vi "Set_Source.vi"(6 "Source Status":T7, 7 "Establish Exp Conditions":bool, 8 "Traverse line":T3 {"Row Duration (mins)" format="%#.1f"; "Row No" min=0; "Trace Gas Concentration (%)" min=0.0 format="%#.2f"; "Emission Rate (l/min)" format="%#.2f"; "Tunnel Speed" format="%#.2f"; "Start X" format="%#.2f"; "Start Y" format="%#.2f"; "Start Z" format="%#.2f"; "End X" format="%#.2f"; "End Y" format="%#.2f"; "End Z" format="%#.2f"; "Averaging time (min)" min=0.0 format="%#.1f"}, 9 "Simulate/Run":T6) -> (0 "Status Cluster":T1, 1 "Flowrates (kg/min)":dbl[](array[numeric]) format="%.2f", 2 "Time Source Started":dbl, 3 "Flowrates Achieved?":bool, 4 "Source requested?":bool, 5 "Source Est Time":dbl format="%.2f")   [LabVIEW 2010]
uses:
  ADAM Client/Sub VIs/ADAM Controls/Client_Source_Status.ctl
  Controls/User_Specific_mode.ctl
  Traverse_cluster.ctl
  Spacing.ctl
  Controls/Multi_run_mode.ctl
  Status_Cluster.ctl
  Multi_Run_Status.ctl
  Globals/Trav_pos_global.vi
  Globals/Extra_Commands_Global.vi
panel:
  # "X           Y            Z"
  # "Start"
  # "End"
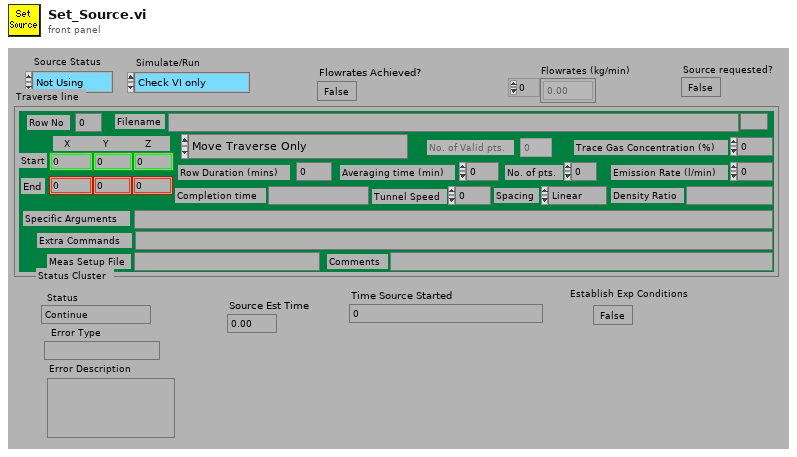
[diagram p1: front panel]
types:
  T1 = typedef "Status_Cluster.ctl" = cluster{"Status":T2, "Error Type":string, "Error Description":string}
  T2 = typedef "Multi_Run_Status.ctl" = enum16{"Continue", "Jump to Next Point", "Jump to Next Row", "Jump To Fall Back", "Terminate Run"}
  T3 = typedef "Traverse_cluster.ctl" = cluster{"Start X":dbl, "Start Y":dbl, "Start Z":dbl, "End X":dbl, "End Y":dbl, "End Z":dbl, "No. of pts.":i32, "Spacing":T4, "Filename":path, "Tunnel Speed":dbl, "Averaging time (min)":dbl, "Extra Commands":string, "Specific Arguments":string, "Emission Rate (l/min)":dbl, "Trace Gas Concentration (%)":dbl, "Density Ratio":string, "Comments":string, "Row No":i32, "Row Type Selector":T5, "Completion time":string, "Row Duration (mins)":dbl, "No. of Valid pts.":i32, "Meas Setup File":string}
  T4 = typedef "Spacing.ctl" = enum16{"Linear", "Log", "Gauss", "Specified", "N/A"}
  T5 = typedef "Multi_run_mode.ctl" = enum16{"Move Traverse Only", "Set Tunnel Speed Only", "Set Source Only", "Set Measurement Conditions", "Single Measurement", "Vertical Profile", "Lateral Profile", "Longitudinal Profile", "Explore Volume", "Multi-Axis Profile", "Auto Calibrate", "Meas Fast FID Bkgnd", "Check Beam Power", "Scanning Valve Measurement", "Run VI Named:", "Set ADAM Ch", "Wait (minutes)", "Send Message", "Synchronize With:", "Fall Back to this Row", "Turn Off Row Repeating", "Blank Row"}
  T6 = typedef "User_Specific_mode.ctl" = enum16{"Check VI only", "Run VI"}
  T7 = typedef "Client_Source_Status.ctl" = enum16{"Not Using", "Using", "Must Have"}
  T8 = cluster{"Emission Rate (l/min)":dbl, "Trace Gas Concentration (%)":dbl, "Density Ratio":string}
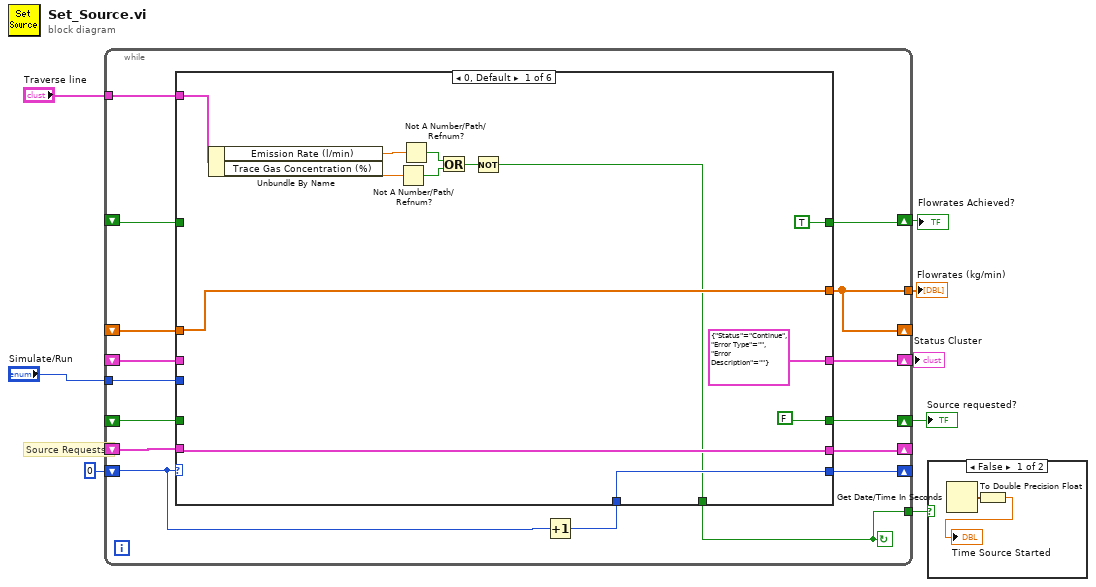
[diagram p0: block diagram]
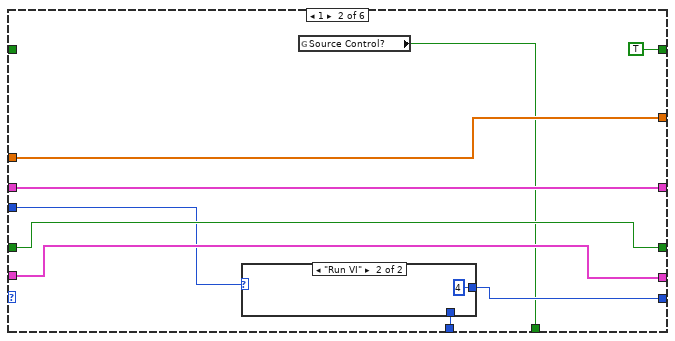
[diagram p3: hidden frame]
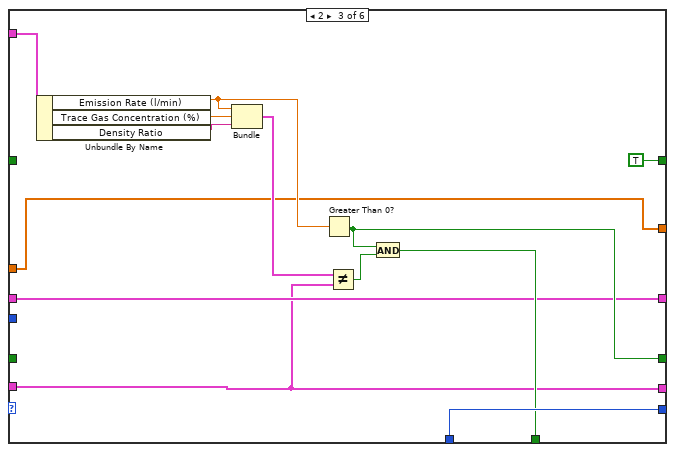
[diagram p5: hidden frame]
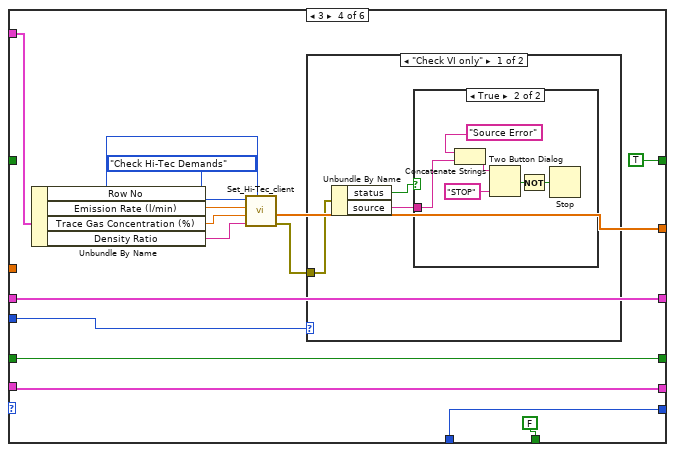
[diagram p6: hidden frame]
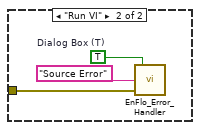
[diagram p8: hidden frame]
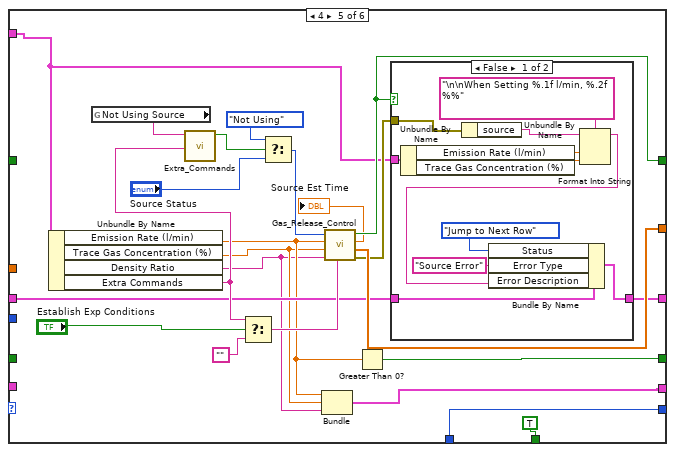
[diagram p9: hidden frame]
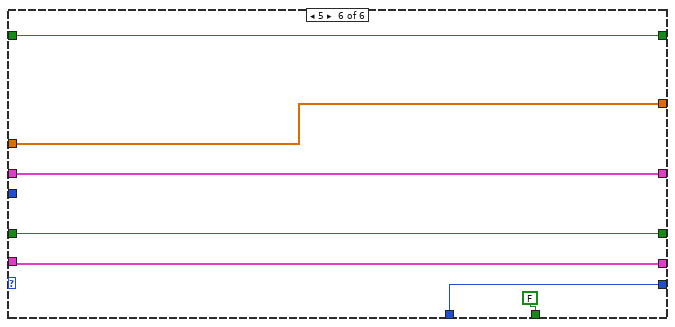
[diagram p11: hidden frame]
diagram:
  # "Source Requests"
  n1 = while {
    shift-left: _ -> [w12]
    shift-right: [w13] -> w4
    shift-left: _ -> [w14]
    shift-right: [w15] -> w5
    shift-left: _ -> [w16]
    shift-right: [w19] -> w6
    shift-left: 0 -> [w18]
    shift-right: [w20] -> _
    shift-left: _ -> [w21]
    shift-right: [w22] -> _
    tunnel: [w22] -> w8
    shift-left: _ -> [w24]
    shift-right: [w23] -> _
    tunnel: "Simulate/Run" -> [w11]
    tunnel: "Traverse line" -> [w10]
    tunnel: [w9] -> w1
    stop <- w9 continue-if-true
    n2 = Increment(x=w18) -> (x+1=w17:i32)
    n3 = case shown="0, Default" w18 {
      tunnel: [w35 w46 w52 w71 w102 w125] -> w22
      tunnel: w24 -> [w32 w44 w50 w68 _ w129]
      tunnel: [w32 w44 w50 w68 w91 w129] -> w23
      tunnel: w21 -> [w35 w46 w52 _ _ w125]
      tunnel: [FALSE w40 w61 w69 w111 w130] -> w19
      tunnel: [TRUE ("Flowrates Achieved?") TRUE ("Flowrates Achieved?") TRUE ("Flowrates Achieved?") TRUE ("Flowrates Achieved?") w103 w124] -> w13
      tunnel: [w25 w38 w55 FALSE TRUE FALSE] -> w9
      tunnel: [w31 w43 w56 w67 w100 w128] -> w20
      tunnel: w17 -> [w31 w41 w56 w67 w100 w128]
      tunnel: w16 -> [_ w40 _ w69 _ w130]
      tunnel: [T1 {"Status"=enum."Continue", "Error Type"="", "Error Description"=""} ("Status Cluster") w42 w51 w65 w101 w126] -> w15
      tunnel: w14 -> [_ w42 w51 w65 w95 w126]
      tunnel: w12 -> [_ _ _ _ _ w124]
      tunnel: w11 -> [_ w39 _ w63 _ _]
      tunnel: w10 -> [w29 _ w49 w62 w89 _]
      frame 0, Default {
        n4 = Unbundle By Name(w29) -> ("Emission Rate (l/min)"=w37:dbl, "Trace Gas Concentration (%)"=w30:dbl)
        n5 = Not A Number/Path/Refnum?(number/path/refnum=w30) -> (NaN/Path/Refnum?=w28:bool)
        n6 = Not A Number/Path/Refnum?(number/path/refnum=w37) -> (NaN/Path/Refnum?=w27:bool)
        n7 = Or(x=w27, y=w28) -> (x .or. y?=w26:bool)
        n8 = Not(x=w26) -> (.not. x?=w25:bool)
      }
      frame 1 {
        n9 = case shown="\"Run VI\"" w39 {
          tunnel: [w47 4] -> w43
          tunnel: w41 -> [w47 _]
          frame "Check VI only" {
          }
          frame "Run VI" {
          }
        }
        n10 = global read "Trav_pos_global.vi" "Source Control?"() -> (w38:bool)
      }
      frame 2 {
        n11 = Unbundle By Name(w49) -> ("Emission Rate (l/min)"=w58:dbl, "Trace Gas Concentration (%)"=w60:dbl, "Density Ratio"=w59:string)
        n12 = Bundle("Emission Rate (l/min)"=w58, "Trace Gas Concentration (%)"=w60, "Density Ratio"=w59) -> (w54:T8)  [unwired: 1 out]
        n13 = Greater Than 0?(x=w58) -> (x > 0?=w61:bool)
        n14 = Not Equal?(x=w54, y=w50) -> (x != y?=w57:bool)
        n15 = And(x=w61, y=w57) -> (x .and. y?=w55:bool)
      }
      frame 3 {
        n16 = Unbundle By Name(w62) -> ("Row No"=w72:i32, "Emission Rate (l/min)"=w75:dbl, "Trace Gas Concentration (%)"=w74:dbl, "Density Ratio"=w73:string)
        n17 = call "Set_Hi-Tec_client.vi"("Row No"=w72, "Density Ratio"=w73, "Strength (% by volume)"=w74, "Stack flowrate (l/min)"=w75, "Mode"=enum16{"Control Hi-Tec", "Check Hi-Tec Demands"}."Check Hi-Tec Demands") -> ("error out"=w64:errorcluster, "Flowrates (kg/min)"=w71:dbl[])  [unwired: 3 out]
        n18 = case shown="\"Check VI only\"" w63 {
          tunnel: w64 -> [w79 w88]
          frame "Check VI only" {
            n19 = Unbundle By Name(w79) -> ("status"=w77:bool, "source"=w78:string)
            n20 = case shown="True" w77 {
              tunnel: w78 -> [_ w84]
              frame False {
              }
              frame True {
                n21 = Concatenate Strings("Source Error" ("Error Type"), w84) -> (w83:string)
                n22 = Two Button Dialog(message=w83, 1:"STOP" ("F button name (\"Cancel\")")) -> (T button?=w81:bool)  [unwired: 1 out]
                n23 = Not(x=w81) -> (.not. x?=w80:bool)
                n24 = Stop(stop? (T)=w80) -> ()
              }
            }
          }
          frame "Run VI" {
            w86 = TRUE  # Dialog Box (T)
            n25 = call "EnFlo_Error_Handler.vi"("error in (no error)"=w88, "Error Type"="Source Error", "Dialog Box (T)"=w86) -> ()  [unwired: 3 out]
          }
        }
      }
      frame 4 {
        n26 = Unbundle By Name(w89) -> ("Emission Rate (l/min)"=w94:dbl, "Trace Gas Concentration (%)"=w93:dbl, "Density Ratio"=w92:string, "Extra Commands"=w105:string)
        n27 = global read "Extra_Commands_Global.vi" "Not Using Source"() -> (w108:string)
        n28 = call "Extra_Commands.vi"("String to Search"=w105, "Command"=w108) -> ("Command Found"=w107:bool)  [unwired: 1 in, 4 out]
        n29 = Select(t=w105, s="Establish Exp Conditions", f="") -> (s? t:f=w104:string)
        n30 = Select(t=Client_Source_Status."Not Using" ("Source Status"), s=w107, f="Source Status") -> (s? t:f=w106:T7)
        n31 = Bundle("Emission Rate (l/min)"=w94, "Trace Gas Concentration (%)"=w93, "Density Ratio"=w92) -> (w91:T8)  [unwired: 1 out]
        n32 = call "Gas_Release_Control.vi"("Extra Commands"=w104, "Density Ratio"=w92, "Strength (% by volume)"=w93, "Stack flowrate (l/min)"=w94, "Source Status"=w106) -> ("error out"=w90:errorcluster, "Flowrates (kg/min)"=w102:dbl[], "Source Est Time (s)"=→"Source Est Time":dbl, "Flowrates Achieved?"=w103:bool)  [unwired: 1 out]
        n33 = Greater Than 0?(x=w94) -> (x > 0?=w111:bool)
        n34 = case shown="False" w103 {
          tunnel: [w118 w123] -> w101
          tunnel: w95 -> [w119 w123]
          tunnel: w89 -> [w114 _]
          tunnel: w90 -> [w113 _]
          frame False {
            n35 = Unbundle By Name(w114) -> ("Emission Rate (l/min)"=w121:dbl, "Trace Gas Concentration (%)"=w120:dbl)
            n36 = Unbundle By Name(w113) -> ("source"=w112:string)
            n37 = Format Into String(format string="\n\nWhen Setting %.1f l/min, %.2f %%" ("Format String"), initial string=w112, w121, w120) -> (resulting string=w115:string)  [unwired: 1 in, 1 out]
            n38 = Bundle By Name(cluster=w119, "Status"=Multi_Run_Status."Jump to Next Row", "Error Type"="Source Error" ("Bundle Element"), "Error Description"=w115) -> (w118:T1)
          }
          frame True {
          }
        }
      }
      frame 5 {
      }
    }
  }
  "Flowrates (kg/min)" <- w8
  "Source requested?" <- w6
  "Flowrates Achieved?" <- w4
  "Status Cluster" <- w5
  n39 = case shown="False" w1 {
    frame False {
      n40 = Get Date/Time In Seconds() -> (seconds since 1Jan1904=w132:timestamp)
      n41 = To Double Precision Float(number=w132) -> (double precision float=→"Time Source Started":dbl)
    }
    frame True {
    }
  }
